vi "RS-232-Core.vi"(0 "VISA resource name":refnum<visa-resource-name>="COM1", 1 "Write to COM Port":bool=TRUE, 3 "String To Write":string="*IDN?", 4 "Read COM Port":bool=TRUE, 5 "baud rate":u32=9600, 6 "Verify CheckSum":bool=TRUE, 9 "Initialize COMPort":bool=TRUE, 11 "Close COMPort":bool=TRUE, 12 "Add CheckSum":bool=TRUE, 15 "bytes to read":u32=5) -> (2 "Sent?":bool, 7 "Close":bool, 8 "CheckSum?":bool, 10 "Response?":bool, 13 "Open?":bool, 14 "Read String":string)   [LabVIEW 2014]
doc: "The Basic Serial Read and Write example performs a Serial Port Read, a Serial Port Write, or a combination of these actions. The user selects the actions (read or write) on the front panel. If both are selected, the VI will write the data first, read data, and then close the VISA session that is opened to the port. This VI will wait until the specified number of bytes is received at the port. Only the number of bytes specified will be read.\n\nINSTRUCTIONS:\n1) Select the serial resource and configuration parameters (baud rate, data bits, parity, stop bits, flow control).\n2) Select the operations to be performed. \n3) Connect the serial port to your device. If no device is available, perform a loopback test by doing one of the following. Short pins 2 and 3 on a RS-232 cable or short pin 4 to pin 8 and pin 5 to pin 9 on a RS-485/422 cable. \n4) Run the VI to see the data read. (The \"read string\" will match the \"string to write\" if a loopback test was performed.)\n\nNote: The parameters set for the serial port must match the parameters of the connected instrument or device. In this example, the bytes to read parameter specifies the number of bytes that the serial port reads. If there were more bytes at the port than the number specified in bytes to read, those bytes would not be read. Also, if you specify to read more bytes than the number of bytes actually read, you might receive a timeout error message.\n\nOn the block diagram, the Configure Serial Port VI sets the configuration parameters. The front panel displays the controls used to configure the basic parameters, such as baud rate, data bits, and parity. Constants configure the other parameters the user probably does not need set. After the VISA Configure Serial Port VI opens the VISA session and configures the port, the VI passes the VISA resource name to other VIs that perform operations on that VISA resource. The VISA Write function sends a command to the serial device and the VISA Read function returns data based on the command. The VISA Close function then closes the reference to the serial device. It is important to close the reference; otherwise communication through with that port through protocols other than VISA might not be possible."
uses:
  <vilib>/Instr/_visa.llb/VISA Configure Serial Port (Instr).vi
panel:
  out "Read Bytes":dbl
  in  "flow control":u16(ring) items=["None"=0, "XON/XOFF"=1, "RTS/CTS"=2, "DTR/DSR"=4]
  in  "stop bits":u16(ring)=10 items=["1.0"=10, "1.5"=15, "2.0"=20]
  in  "parity":u16(ring) items=["None", "Odd", "Even", "Mark", "Space"]
  in  "data bits":u16=8 min=5 max=8 step=1
  # "Select the serial resource and the operations (Read, Write, or both) to be performed.  If both are selected, the VI will write the data first, read data and then close the VISA session that is opened to the port.  This VI will wait until the specified number of bytes is received at the port. Only the number of bytes specified will be read."
  # "For additional information select File >> VI Properties >> Documentation"
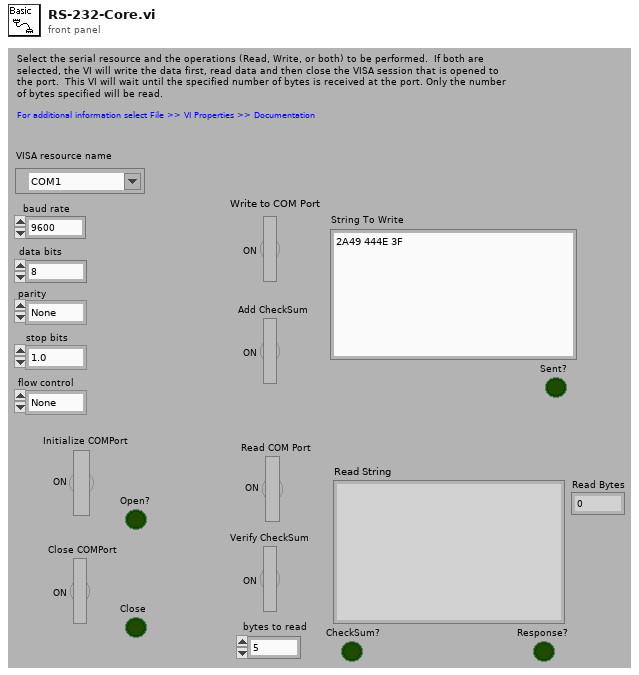
[diagram p1: front panel]
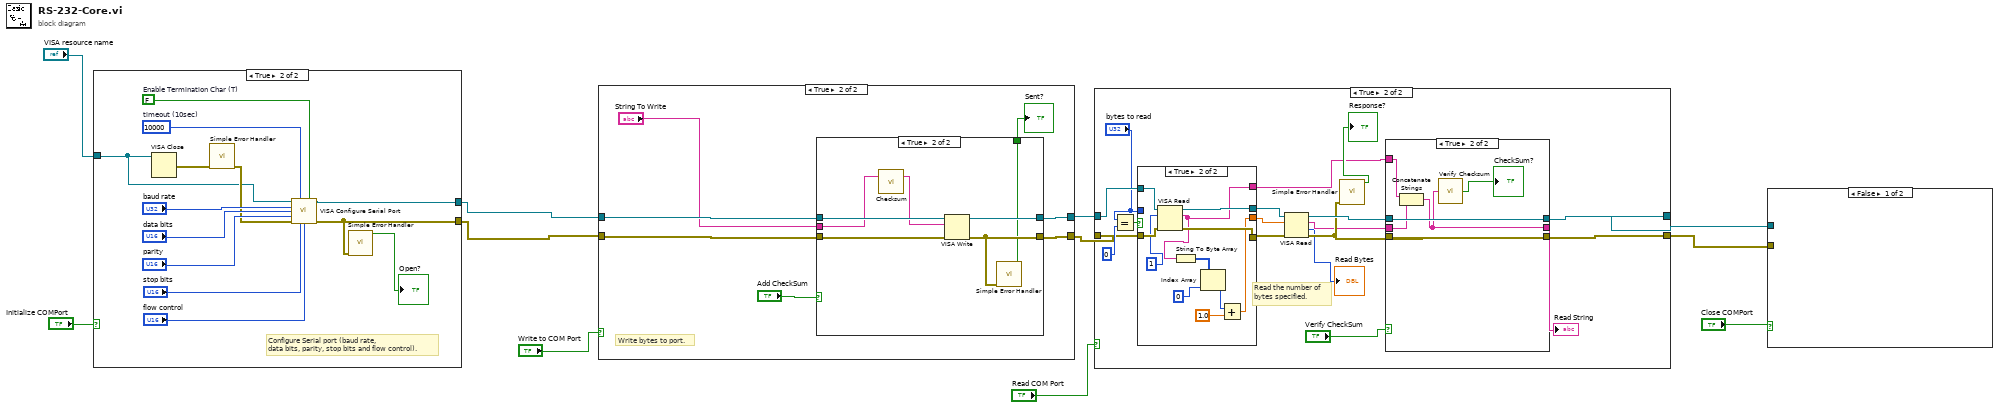
[diagram p0: block diagram]
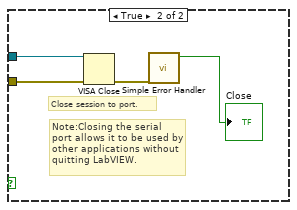
[diagram p2: hidden frame]
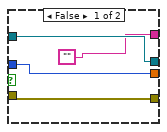
[diagram p4: hidden frame]
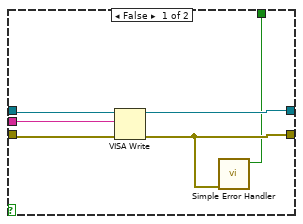
[diagram p7: hidden frame]
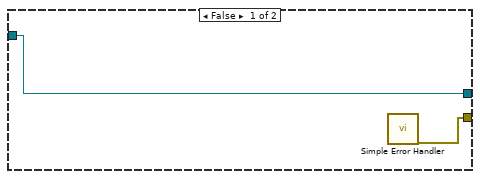
[diagram p8: hidden frame]
diagram:
  n1 = case shown="True" "Initialize COMPort" {
    tunnel: "VISA resource name" -> [w13 w16]
    tunnel: [w13 w19] -> w2
    tunnel: [w12 w15] -> w1
    frame False {
      n2 = call <vilib>:"Simple Error Handler.vi"() -> ("error out"=w12:errorcluster)  [unwired: 5 in, 4 out]
    }
    frame True {
      w23 = FALSE  # Enable Termination Char (T)
      w24 = u32 10000  # timeout (10sec)
      # "Configure Serial port (baud rate,\ndata bits, parity, stop bits and flow control)."
      n3 = VISA Close(VISA resource name=w16) -> (error out=w18:errorcluster)  [unwired: 1 in]
      n4 = call <vilib>:"Simple Error Handler.vi"("error in (no error)"=w18) -> ("error out"=w17:errorcluster)  [unwired: 4 in, 4 out]
      n5 = call-poly "VISA Configure Serial Port"("VISA resource name"=w16, "timeout (10sec)"=w24, "Enable Termination\nChar (T)"=w23, "baud rate (9600)"="baud rate", "data bits (8)"="data bits", "parity (0:none)"="parity", "error in (no error)"=w17, "stop bits (10: 1 bit)"="stop bits", "flow control (0:none)"="flow control") -> ("VISA resource name out"=w19:refnum<visa-resource-name>, "error out"=w15:errorcluster)  [unwired: 5 in]
      n6 = call <vilib>:"Simple Error Handler.vi"("error in (no error)"=w15) -> ("error?"=→"Open?":bool)  [unwired: 4 in, 4 out]
    }
  }
  n7 = case shown="True" "Write to COM Port" {
    tunnel: [w28 w35] -> w3
    tunnel: w2 -> [w27 w34]
    tunnel: w1 -> [w28 w33]
    tunnel: [w27 w32] -> w4
    frame False {
    }
    frame True {
      # "Write bytes to port."
      n8 = case shown="True" "Add CheckSum" {
        tunnel: [w37 w45] -> w35
        tunnel: w34 -> [w40 w48]
        tunnel: w33 -> [w39 w47]
        tunnel: [w41 w46] -> w32
        tunnel: "String To Write" -> [w38 w43]
        tunnel: [w36 w44] -> w29
        frame False {
          n9 = VISA Write(VISA resource name=w40, write buffer=w38, error in (no error)=w39) -> (VISA resource name out=w41:refnum<visa-resource-name>, error out=w37:errorcluster)  [unwired: 1 out]
          n10 = call <vilib>:"Simple Error Handler.vi"("error in (no error)"=w37) -> ("error?"=w36:bool)  [unwired: 4 in, 4 out]
        }
        frame True {
          n11 = call "Checksum.vi"("HEX String to Calculate CheckSum"=w43) -> ("Hex String with CheckSum"=w42:string)  [unwired: 2 out]
          n12 = VISA Write(VISA resource name=w48, write buffer=w42, error in (no error)=w47) -> (VISA resource name out=w46:refnum<visa-resource-name>, error out=w45:errorcluster)  [unwired: 1 out]
          n13 = call <vilib>:"Simple Error Handler.vi"("error in (no error)"=w45) -> ("error?"=w44:bool)  [unwired: 4 in, 4 out]
        }
      }
      "Sent?" <- w29
    }
  }
  n14 = case shown="True" "Read COM Port" {
    tunnel: w3 -> [w50 w56]
    tunnel: [w50 w64] -> w5
    tunnel: [w49 w66] -> w6
    tunnel: w4 -> [w49 w57]
    frame False {
    }
    frame True {
      # "Read the number of bytes specified."
      n15 = Equal?(x="bytes to read", y=u32 0) -> (x = y?=w59:bool)
      n16 = case shown="True" w59 {
        tunnel: w57 -> [w71 w83]
        tunnel: w56 -> [w70 w82]
        tunnel: [w70 w81] -> w52
        tunnel: [w71 w80] -> w55
        tunnel: "bytes to read" -> [w72 _]
        tunnel: [w72 w74] -> w53
        tunnel: ["" w73] -> w51
        frame False {
        }
        frame True {
          n17 = VISA Read(VISA resource name=w83, byte count=u32 1, error in (no error)=w82) -> (VISA resource name out=w80:refnum<visa-resource-name>, read buffer=w73:string, error out=w81:errorcluster)  [unwired: 1 out]
          n18 = String To Byte Array(string=w73) -> (unsigned byte array=w78:u8[])
          n19 = Index Array(array=w78, index=0) -> (element=w75:u8)
          n20 = Add(x=w75, y=1.0) -> (x+y=w74:dbl)
        }
      }
      n21 = VISA Read(VISA resource name=w55, byte count=w53, error in (no error)=w52) -> (VISA resource name out=w67:refnum<visa-resource-name>, read buffer=w63:string, return count=→"Read Bytes":u32, error out=w65:errorcluster)
      n22 = call <vilib>:"Simple Error Handler.vi"("error in (no error)"=w65) -> ("error?"=→"Response?":bool)  [unwired: 4 in, 4 out]
      n23 = case shown="True" "Verify CheckSum" {
        tunnel: w67 -> [w86 w92]
        tunnel: [w86 w92] -> w66
        tunnel: w65 -> [w85 w91]
        tunnel: [w85 w91] -> w64
        tunnel: w63 -> [w84 w88]
        tunnel: [w84 w87] -> w62
        tunnel: w51 -> [_ w89]
        frame False {
        }
        frame True {
          n24 = Concatenate Strings(w89, w88) -> (w87:string)
          n25 = call "Verify Checksum.vi"("HEX String to Verify CheckSum"=w87) -> ("CheckSum OK"=→"CheckSum?":bool)
        }
      }
      "Read String" <- w62
    }
  }
  n26 = case shown="False" "Close COMPort" {
    tunnel: w5 -> [_ w96]
    tunnel: w6 -> [_ w95]
    frame False {
    }
    frame True {
      # "Note:Closing the serial port allows it to be used by other applications without\nquitting LabVIEW."
      # "Close session to port."
      n27 = VISA Close(VISA resource name=w95, error in (no error)=w96) -> (error out=w94:errorcluster)
      n28 = call <vilib>:"Simple Error Handler.vi"("error in (no error)"=w94) -> ("error?"=→"Close":bool)  [unwired: 4 in, 4 out]
    }
  }
